vi "Main Server Process Loop.vi"(11 "Base Server in":refnum<class "Server.lvclass">) -> ()   [LabVIEW 2024, in "Ramses Framework.lvlib" / "Server.lvclass"]
uses:
  Server.lvclass
  <vilib>/MediaMongrels Ltd/WebSockets/Sockets/Socket Listener/Socket Listener.lvclass
  Handler/Handler.lvclass
  <vilib>/MediaMongrels Ltd/WebSockets/WebSockets/WebSocket Server/WebSocket Server.lvclass
  C:/Program Files (x86)/National Instruments/LabVIEW 2024/vi.lib/MediaMongrels Ltd/WebSockets/WebSockets/WebSocket/WebSocket.lvclass
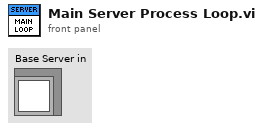
[diagram p1: front panel]
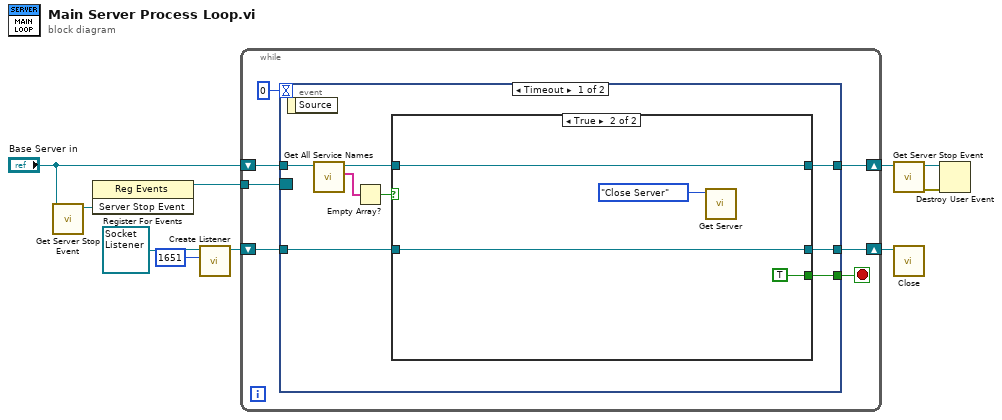
[diagram p0: block diagram]
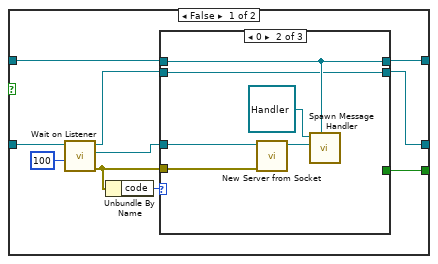
[diagram p2: hidden frame]
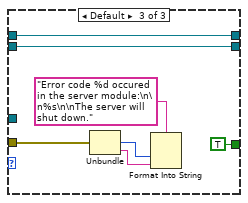
[diagram p4: hidden frame]
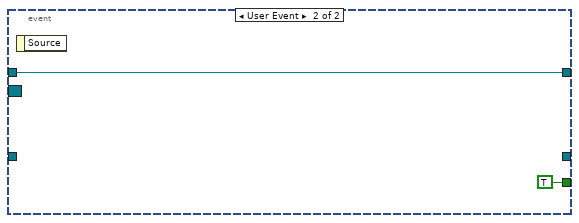
[diagram p5: hidden frame]
diagram:
  n1 = call-dynamic "Get Server Stop Event.vi"("Base Server in"="Base Server in") -> ("Server Stop Event"=w9:refnum<user-event>)  [unwired: 9 in, 1 out]
  n2 = register-events(w9) -> (reference out=w8:refnum<event-registration>)  [unwired: 2 in, 1 out]
  n3 = call-dynamic "Create Listener.vi"("Port"=u16 1651 ("timeout ms (wait forever: -1)"), "Socket Listener in"=refnum<class "Socket Listener.lvclass"> refnum) -> ("Socket Listener out"=w5:refnum<class "Socket Listener.lvclass">)  [unwired: 8 in, 1 out]
  n4 = while {
    shift-right: [w15] -> w10
    shift-left: "Base Server in" -> [w17]
    tunnel: w8 -> [w16]
    shift-right: [w11] -> w4
    shift-left: w5 -> [w12]
    stop <- w14 stop-if-true
    n5 = event shown="[0] Timeout" {
      selector: w16 -> [_ _]
      dyn-events: _ -> [_ _]
      timeout: 0 -> [_ _]
      tunnel: w17 -> [w20 w56]
      tunnel: [w25 w56] -> w15
      tunnel: [w24 TRUE] -> w14
      tunnel: w12 -> [w23 _]
      tunnel: [w22 _] -> w11
      event Timeout {
        n6 = event-data() -> ()  [unwired: 1 in, 1 out]
        n7 = call-dynamic "Get All Service Names.vi"("Server in"=w20) -> ("Service Names"=w19:string[], "Server out"=w21:refnum<class "Server.lvclass">)  [unwired: 8 in, 1 out]
        n8 = Empty Array?(array=w19) -> (empty?=w18:bool)
        n9 = case shown="True" w18 {
          tunnel: [w35 w54] -> w25
          tunnel: [w34 TRUE] -> w24
          tunnel: w23 -> [w32 w53]
          tunnel: [w27 w53] -> w22
          tunnel: w21 -> [w26 w54]
          frame False {
            n10 = call-dynamic "Wait on Listener.vi"("timeout ms (5000)"=100 ("timeout ms (wait forever: -1)"), "Socket Listener in"=w32) -> ("error out"=w29:errorcluster, "Socket out"=w30:refnum<class "Socket.lvclass">, "Socket Listener out"=w28:refnum<class "Socket Listener.lvclass">)  [unwired: 7 in]
            n11 = Unbundle By Name(w29) -> ("code"=w33:i32)
            n12 = case shown="0" w33 {
              tunnel: w26 -> [w37 w43 w50]
              tunnel: [w37 w43 w50] -> w35
              tunnel: [_ _ TRUE] -> w34
              tunnel: w29 -> [_ w41 w45]
              tunnel: w30 -> [_ w40 _]
              tunnel: w28 -> [w36 w38 w44]
              tunnel: [w36 w38 w44] -> w27
              frame 56 {
              }
              frame 0 {
                n13 = call <vilib>:"New Server from Socket.vi"("error in (no error)"=w41, "Socket"=w40) -> ("WebSocket Server out"=w39:refnum<class "WebSocket Server.lvclass">)  [unwired: 8 in, 1 out]
                n14 = call "Spawn Message Handler.vi"("Base Server"=w43, "WebSocket in"=w39, "Message Handler in"=refnum<class "Handler.lvclass"> refnum ("Handler.lvclass")) -> ()  [unwired: 8 in, 1 out]
              }
              frame Default {
                n15 = Unbundle(w45) -> ("code"=w46:i32, "source"=w47:string)  [unwired: 1 out]
                n16 = Format Into String(format string="Error code %d occured in the server module:\n\n%s\n\nThe server will shut down.", w46, w47) -> ()  [unwired: 2 in, 2 out]
              }
            }
          }
          frame True {
            n17 = call "Get Server.vi"("Method"=enum16{"Get Server", "Close Server"}."Close Server") -> ()  [unwired: 9 in, 2 out]
          }
        }
      }
      event User Event {
        n18 = event-data() -> ()  [unwired: 1 in, 1 out]
      }
    }
  }
  n19 = call-dynamic "Get Server Stop Event.vi"("Base Server in"=w10) -> ("error out"=w2:errorcluster, "Server Stop Event"=w1:refnum<user-event>)  [unwired: 9 in]
  n20 = call-dynamic "Close.vi"("Socket Listener in"=w4) -> ()  [unwired: 10 in, 1 out]
  n21 = Destroy User Event(user event=w1, error in=w2) -> ()  [unwired: 1 out]
